vi "Dashboard Main.vi"() -> ()   [LabVIEW 2018]
uses:
  Subsystems/Drive/MotionProfile/StartingPosition.ctl
  Subsystems/Drive/MotionProfile/Path_Decider.ctl
  <vilib>/Utility/miscctls.llb/LVRowAndColumnTypeDef.ctl
  <vilib>/event_ctls.llb/eventvkey.ctl
  <vilib>/Rock Robotics/Network Tables/NT Read Numeric Array.vi
  <vilib>/Rock Robotics/WPI/Dashboard/WPI_DashboardLogging Global.vi
panel:
  in  "Select Auto":string(combo)="Select Autonomous ..."
  out "NT Connection":bool
  out "Camera Perf":string
  in  "Camera Settings":T1={"Frame Rate"=30, "Compression"=30, "Size"=1, "DB Camera Config"=FALSE} {"Frame Rate" scale=1.0..30.0; "Compression" scale=100.0..-1.0; "Size" items=["640x480", "320x240", "160x120"]}
  in  "TCP":refnum<k5>
  out "Robot IP":string
  out "Image Message":string="Timeout in Camera Communications"
  in  "Dashboard Tab":T2(tab)
  out "Mode":T3(ring)=enum."Auto Disabled"
  out "Right Camera Perf":cluster{"Bandwidth (Mbps)":dbl, "FPS":dbl}
  out "Yaw":dbl(graph)
  out "Pitch":dbl(graph)
  out "Roll":dbl(graph)
  out "climbPoweredIRLeft":bool
  out "lineIRRearLeft":bool
  out "climbPoweredIRRight":bool
  out "climbSkidIRRight":bool
  out "climbSkidIRLeft":bool
  out "lineIRFrontLeft":bool
  out "lineIRRearRight":bool
  out "lineIRFrontRight":bool
  out "ClimbRearPosition":dbl
  out "ClimbFrontPosition":dbl
  out "DriveLeftEncoder":dbl
  out "DriveRightEncoder":dbl
  out "HatchPanelDistance":dbl(graph)
  out "DriveIMU":T4(graph)
  out "Sonar":dbl(graph)
  in  "Auto Options":T7={"Starting Position"=enum."Middle L1", "First Score Pos"=enum."7", "Second Score Pos"=enum."5"}
  out "AutoValid?":bool
  in  "Rec Mode":enum32{"Stop", "Record", "Playback"}(radio)
  in  "Camera Settings Right":T1={"Frame Rate"=30, "Compression"=30, "Size"=1, "DB Camera Config"=FALSE} {"Frame Rate" scale=1.0..30.0; "Compression" scale=100.0..-1.0; "Size" items=["640x480", "320x240", "160x120"]}
  in  "Camera Name Right":string(combo)="No Camera Selection"
  out "HatchPanelSwitchA":bool
  out "HatchPanelSwitchB":bool
  out "Match Number":dbl
  out "Replay Number":dbl
  out "Match Type":string
  out "Competion":string
  out "Camera Image Right":T8(plugin-control)
  out "Camera Image":T8(plugin-control)
  in  "DB/String 9":string
  in  "DB/String 8":string
  in  "DB/String 7":string
  in  "DB/String 6":string
  in  "DB/String 5":string
  in  "DB/String 4":string
  in  "DB/String 3":string
  in  "DB/String 2":string
  in  "DB/String 1":string
  in  "DB/String 0":string
  in  "DB/Slider 0":dbl(slide) scale=0.0..5.0
  in  "DB/Slider 1":dbl(slide) scale=0.0..5.0
  in  "DB/Slider 2":dbl(slide) scale=0.0..5.0
  in  "DB/Slider 3":dbl(slide) scale=0.0..5.0
  out "DB/LED 3":bool
  out "DB/LED 2":bool
  out "DB/LED 1":bool
  out "DB/LED 0":bool
  in  "DB/Button 3":bool
  in  "DB/Button 2":bool
  in  "DB/Button 1":bool
  in  "DB/Button 0":bool caption="New Name"
  in  "A PID gains":T9={"proportional gain (Kc)"=0.039, "integral time (Ti, min)"=0.0, "derivative time (Td, min)"=0.0018000000000000004} {"derivative time (Td, min)" format="%.4f"; "integral time (Ti, min)" format="%.4f"; "proportional gain (Kc)" format="%.4f"}
  in  "B PID gains":T9={"proportional gain (Kc)"=0.027999999999999997, "integral time (Ti, min)"=0.0, "derivative time (Td, min)"=0.0018000000000000004} {"derivative time (Td, min)" format="%.4f"; "integral time (Ti, min)" format="%.4f"; "proportional gain (Kc)" format="%.4f"}
  in  "Test Slider":dbl(slide) scale=0.0..100.0 scale format="%#_3g"
  in  "On/Off":bool caption="Solenoid"
  in  "Test Name":u16(ring) items=["Select the test to run..."]
  in  "Test Tree":string(tree)
  in  "Motor":cluster{"Value":dbl, "Enable":bool} {"Value" scale=-1.0..1.0 scale format="%#_3g"}
  out "Progress":T10 {"Test Progress" scale=0.0..100.0}
  in  "Rev/Fwd":cluster{"Forward":bool, "Reverse":bool}
  in  "Test Ring":u16(ring) items=["Monochrome", "Color"]
  out "Cmd Status":string
  in  "Execute Command":bool
  in  "Command Params":string[][](table)
  in  "Command Selection":i32(listbox)
  in  "CheckList":i32(listbox)
  out "Tree":string(tree)
  out "Background":bool
  in  "Camera Name":string(combo)="No Camera Selection"
  # "HW"
  # "HW"
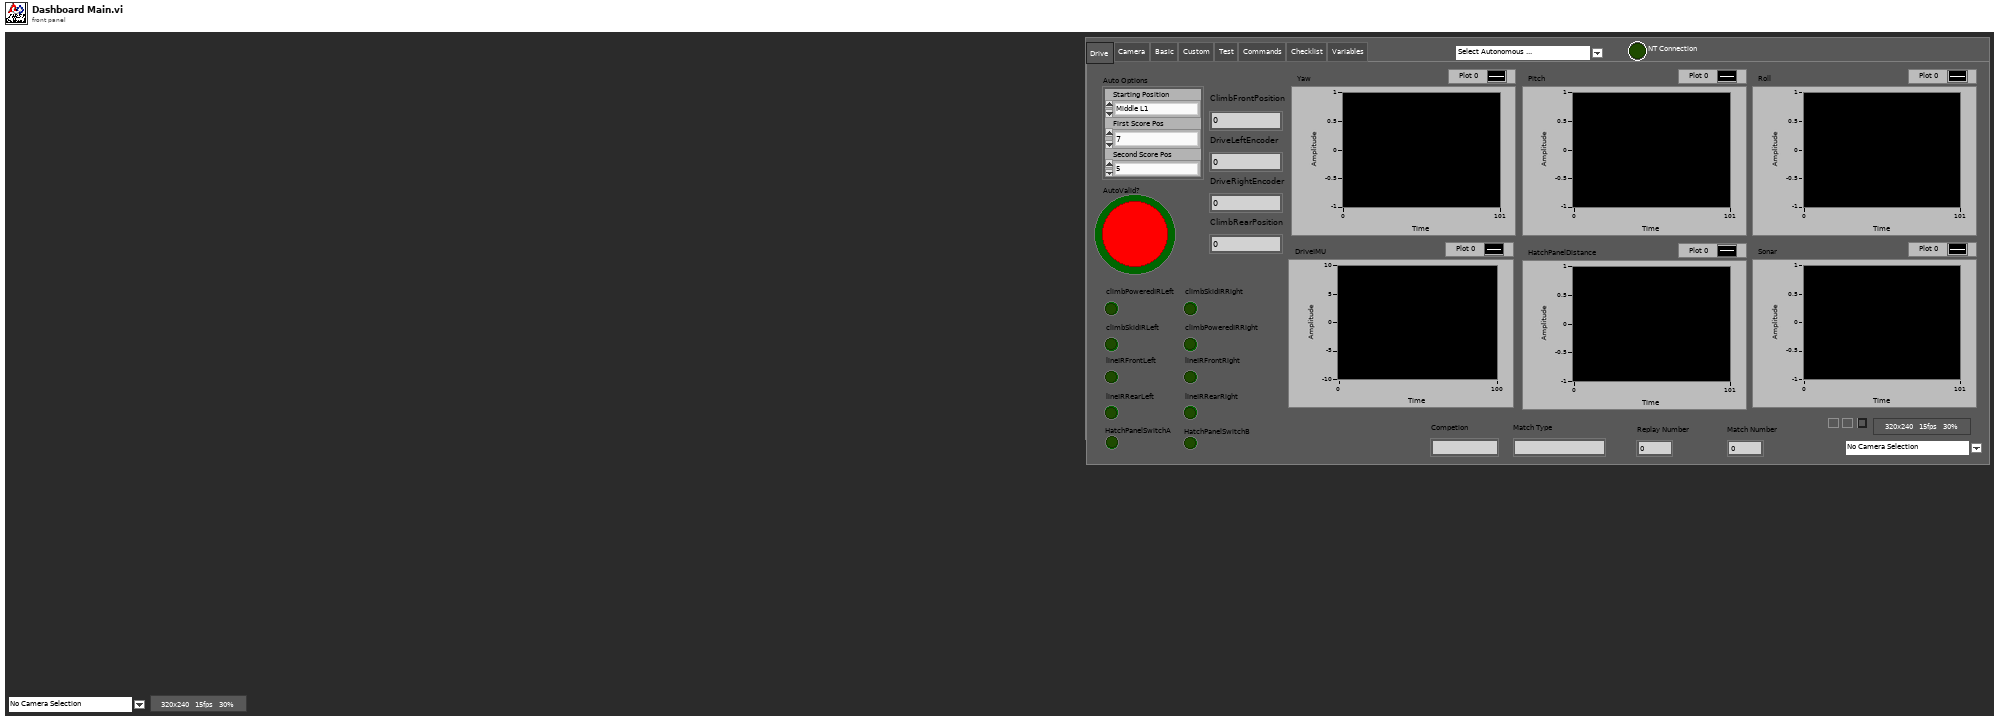
[diagram p1: front panel]
types:
  T1 = cluster{"Frame Rate":i32, "Compression":i32, "Size":u16, "DB Camera Config":bool}
  T2 = enum32{"Drive", "Camera", "Basic", "Custom", "Test", "Commands", "Checklist", "Variables"}
  T3 = enum8{"Tele-Op Disabled", "Tele-Op Enabled", "Auto Disabled", "Auto Enabled", "Test Disabled", "Test Enabled", "Disconnected", "No Code", "E-Stop"}
  T4 = cluster{"Numeric":dbl, "Numeric":dbl, "Numeric":dbl}
  T5 = typedef "StartingPosition.ctl" = enum16{"Left L1 ", "Middle L1", "Right L1", "Left L2", "Right L2", "Don't Move"}
  T6 = typedef "Path_Decider.ctl" = enum16{"1", "2", "3", "4", "5", "6", "7", "8", "Left_Rocket_Front", "Left_Rocket_Rear", "Right_Rocket_Front", "Right_Rocket_Rear"}
  T7 = cluster{"Starting Position":T5, "First Score Pos":T6, "Second Score Pos":T6}
  T8 = typedef "IMAQ Image.ctl" = refnum<image>
  T9 = cluster{"proportional gain (Kc)":dbl, "integral time (Ti, min)":dbl, "derivative time (Td, min)":dbl}
  T10 = cluster{"Test Progress":u8, "Test Progress Text":string}
  T11 = cluster{"Save Path":path, "Interval (s)":dbl, "Keep":i32}
  T12 = typedef "Image Type" = u32
  T13 = cluster{"IDs":cluster{"RPC field ID":u16, "Unique ID":u16}, "String":string}
  T14 = cluster{"Error Strings":string, "Disable Counts":cluster{u16, u16}, "Rail Faults":cluster{u16, u16, u16}, "Robot IP":string, "DB Mode":u8, "Event Info":cluster{"Name":string, "Type":u8, "Number":u16, "Replay":u8}}
  T15 = cluster{"Storage":cluster{"Disk Free":u64, "RAM Block":u32, "RAM free":u32}, "CPU Utilization":cluster{"CPU % ISR":sgl, "CPU % Time Crit":sgl, "CPU % Timed Str":sgl, "CPU % High":sgl, "CPU % Above":sgl, "CPU % Normal":sgl, "CPU % Low":sgl}, "CAN":cluster{"% Bus Utilization":sgl, "Bus Off Cnt":u32, "TX_FIFO Full Cnt":u32, "Receive Error Cnt":u8, "Transmit Error Cnt":u8}, "HID":cluster{"HID Outputs":u32, "Rumble Low":u16, "Rumble High":u16}[]}
  T16 = cluster{"Status bits":cluster{"Test Mode":bool, "Autonomous":bool, "Enabled":bool, "Code Start":bool, "Brownout":bool, "Reserved 2":bool, "Reserved 3":bool, "E-Stop":bool}, "Code Trace":cluster{"Disabled":bool, "TeleOp":bool, "Auto":bool, "Test":bool}, "Controller Type":enum16{"unknown", "cRIO", "roboRio"}, "Code?":enum16{"unknown", "noCode", "code"}, "Battery V":dbl}
  T17 = cluster{"Control Bits":cluster{"TestMode":bool, "Autonomous":bool, "Enabled":bool, "FMS Present":bool, bool, bool, bool, "E-Stop":bool}, "Team Station ":u8, "Countdown":sgl, "Joystick Values":cluster{"Axes":dbl[], "Buttons":bool[], "POVs":i16[]}[]}
  T18 = cluster{"Axes":dbl[], "Buttons":bool[], "POVs":i16[]}[]
  T19 = cluster{"Axes":dbl[], "Buttons":bool[], "POVs":i16[]}
  T20 = cluster{"Camera Image":refnum<vi>, "Dashboard Tab":refnum<vi>, "Background":refnum<vi>, "Rec Mode":refnum<vi>, "Test Slider":refnum<vi>, "On/Off ":refnum<vi>, "Test Ring":refnum<vi>, "Rev/Fwd":refnum<vi>, "Test Name":refnum<vi>, "Motor":refnum<vi>, "Progress":refnum<vi>, "CheckList":refnum<vi>, "Tree":refnum<vi>, "Test Tree":refnum<vi>, "Command Params":refnum<vi>, "Command Selection":refnum<vi>, "Execute Command":refnum<vi>, "Cmd Status":refnum<vi>, "Camera Settings":refnum<vi>, "Camera Name":refnum<vi>, "Camera Perf":refnum<vi>, "Camera Settings Right":refnum<vi>, "Camera Name Right":refnum<vi>, "Camera Image Right":refnum<vi>}
  T21 = cluster{"Global Rectangle":i32[], "Contours":cluster{"Contour Type":u32, "ROI Type":u32, "Points":i32[]}[]}
  T22 = cluster{"Camera Name":string, string, "Saved DB Images Info":cluster{"Save Path":path, "Interval (s)":dbl, "Keep":i32}}
  T23 = cluster{"Camera Name Right":string, string, "Saved DB Images Info":cluster{"Save Path":path, "Interval (s)":dbl, "Keep":i32}}
  T24 = cluster{"Operation":enum16{"Update", "Clear"}, "Color Box":u32}[]
  T25 = typedef "eventvkey.ctl" = enum16{"ASCII", "Enter", "Return", "Shift", "Ctrl", "Alt", "Cmd", "Opt", "Caps", "NumLock", "Clear", "Break", "Up", "Down", "Left", "Right", "Insert", "Delete", "Home", "End", "PageUp", "PageDown", "Escape", "Help", "Pause", "ScrollLock", "F1", "F2", "F3", "F4", "F5", "F6", "F7", "F8", "F9", "F10", "F11", "F12", "F13", "F14", "F15", "F16", "F17", "F18", "F19", "F20", "F21", "F22", "F23", "F24", "Play", "VolumeUp", "VolumeDown", "Mute", "Two Byte Char"}
  T26 = cluster{"Image Size":bool, "Image Type":bool, "Pixel Value":bool, "ROI Information":bool, "Zoom Factor":bool}
  T27 = cluster{"Operation":enum16{"Update", "Clear"}, "Color Box":u32}
  T28 = typedef "LVRowAndColumnTypeDef.ctl" = cluster{"Row":i32, "Column":i32}
  T29 = cluster{"Shift":bool, "Ctrl":bool, "Alt":bool, "Cmd":bool, "Opt":bool}
  T30 = cluster{"Yaw":dbl, "DriveIMU":cluster{"Numeric":dbl, "Numeric":dbl, "Numeric":dbl}, "Sonar":dbl, "Pitch":dbl, "Roll":dbl, "HatchPanelDistance":dbl, "HatchPanelDetect":bool, "climbPoweredIRRight":bool, "climbPoweredIRLeft":bool, "climbSkidIRLeft":bool, "climbSkidIRRight":bool, "lineIRFrontLeft":bool, "lineIRFrontRight":bool, "lineIRRearLeft":bool, "lineIRRearRight":bool, "ClimbFrontPosition":dbl, "ClimbRearPosition":dbl, "DriveRightEncoder":dbl, "DriveLeftEncoder":dbl, "HatchPanelSwitchA":bool, "HatchPanelSwitchB":bool}
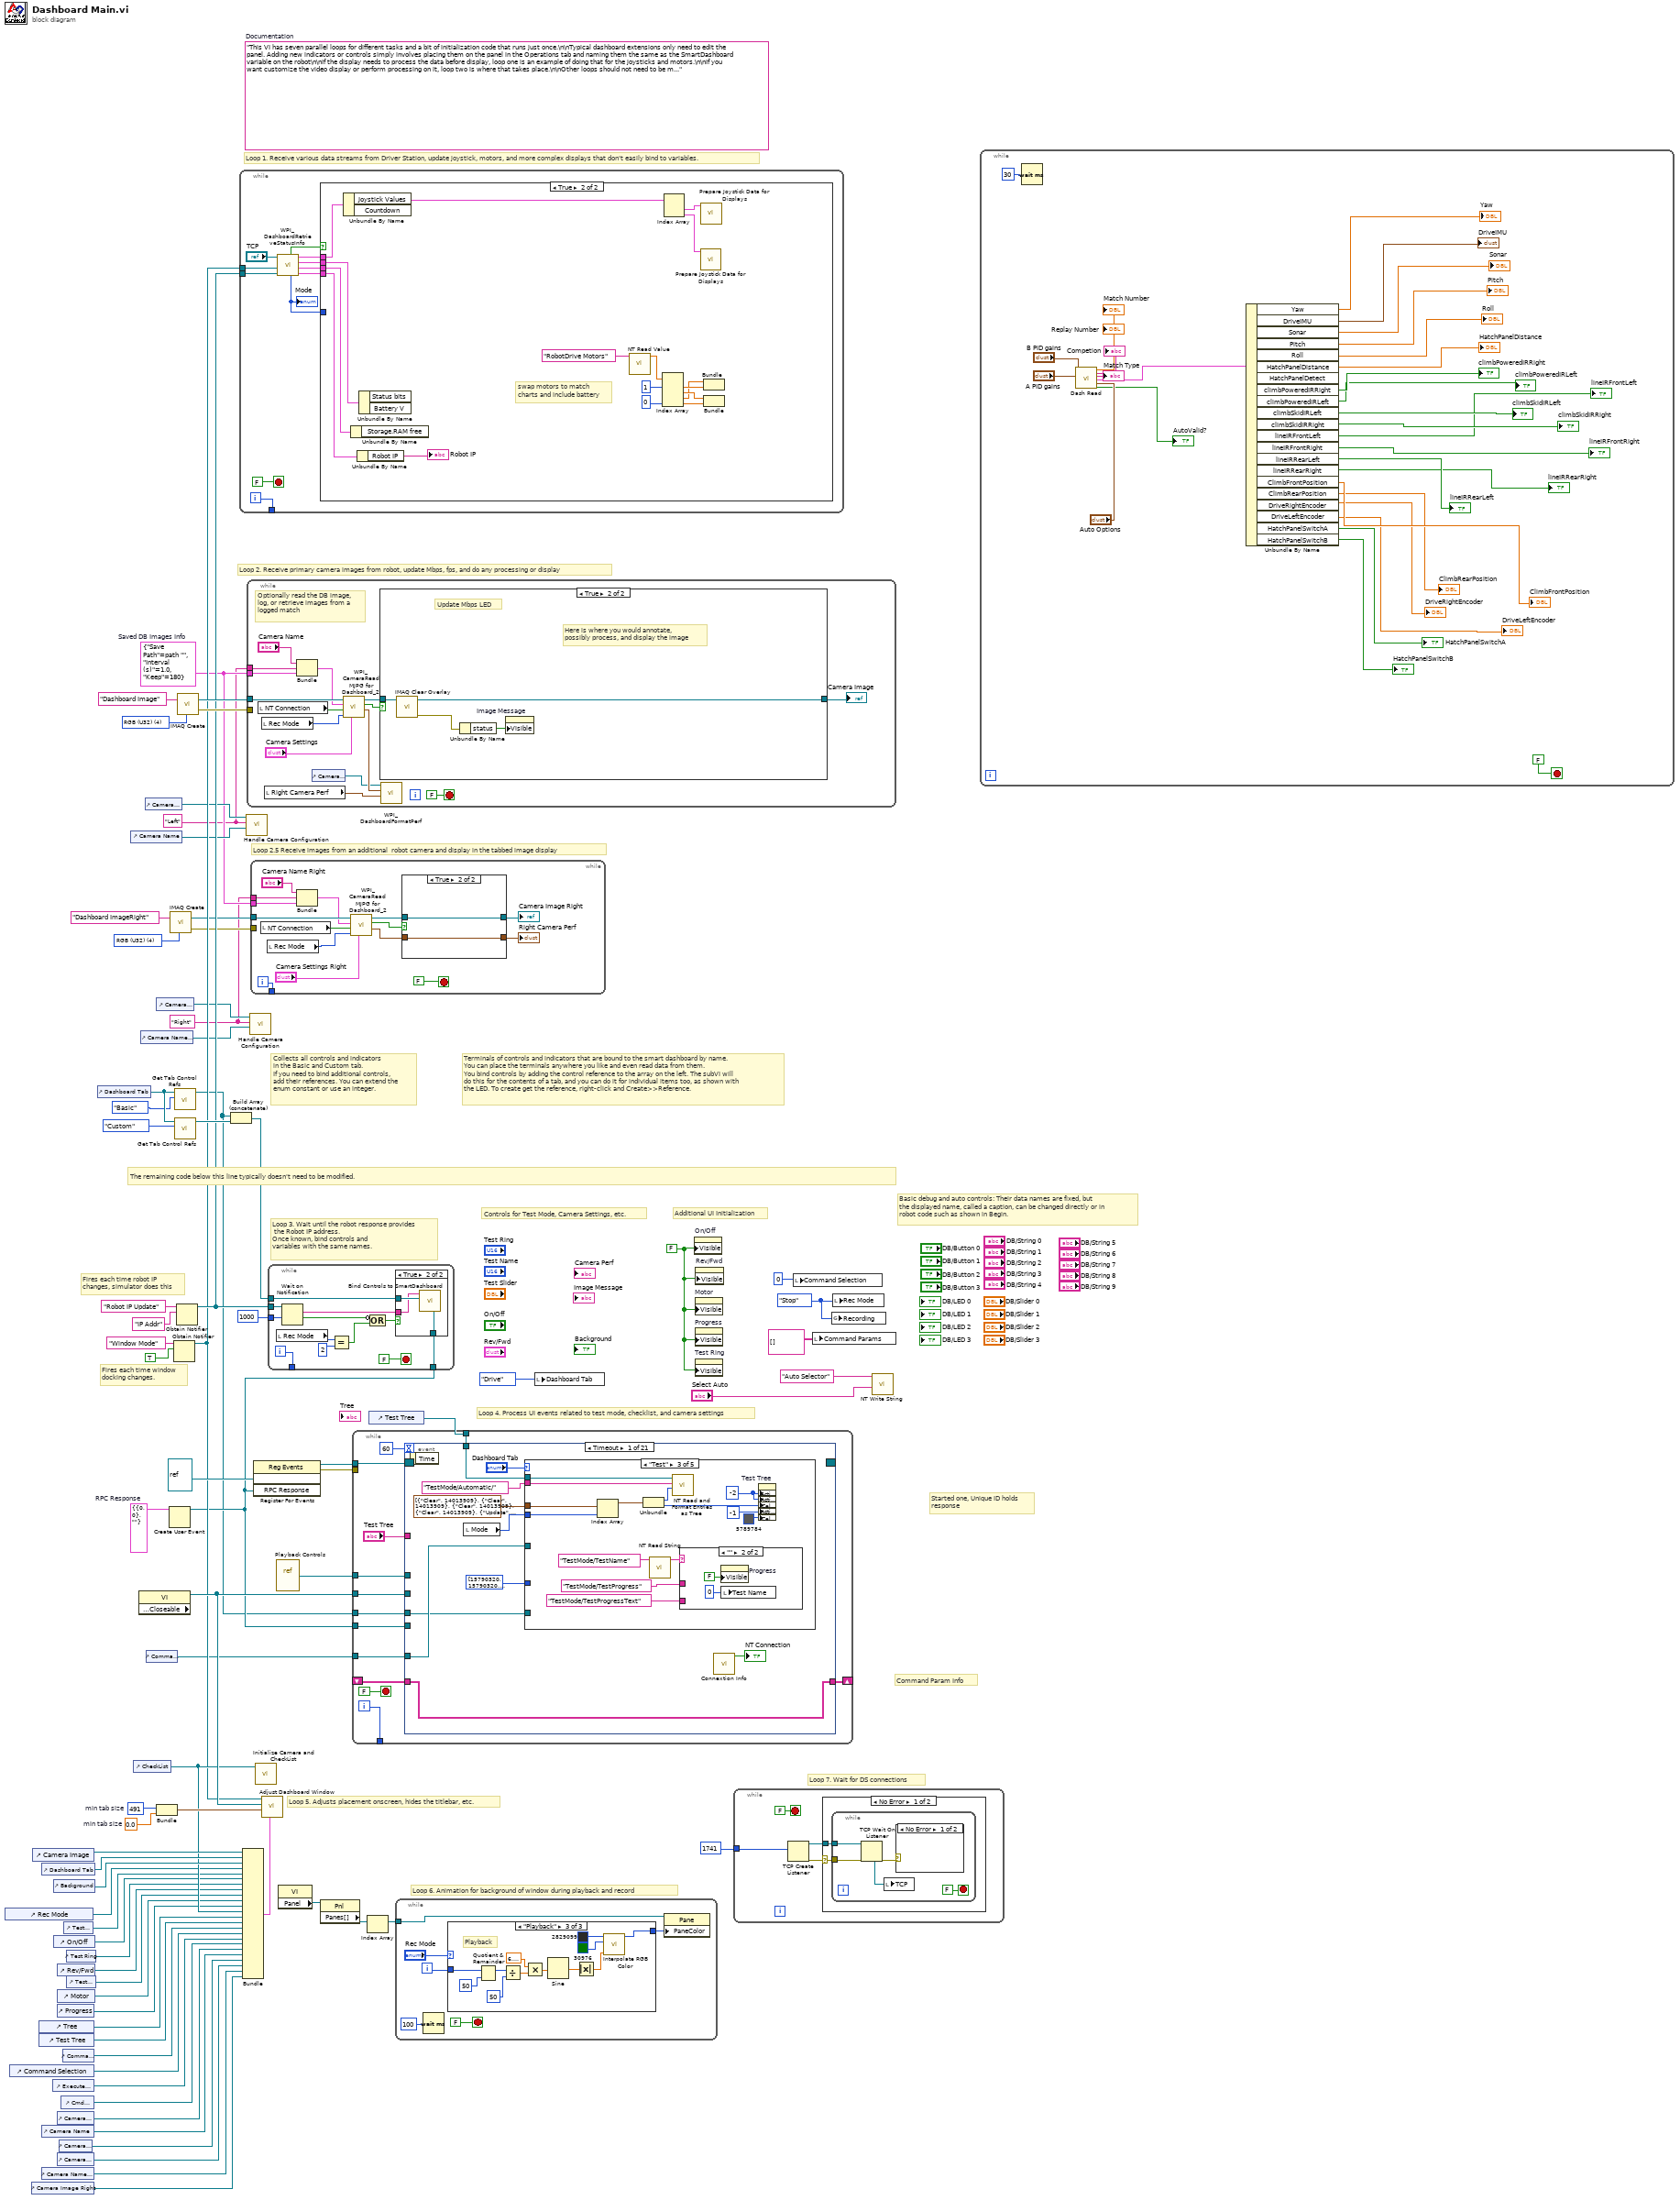
[diagram p0: block diagram]
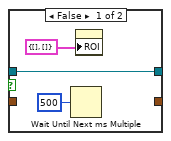
[diagram p2: hidden frame]
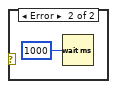
[diagram p3: hidden frame]
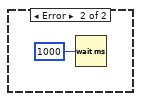
[diagram p4: hidden frame]
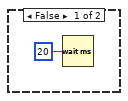
[diagram p5: hidden frame]
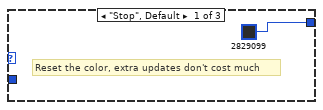
[diagram p6: hidden frame]
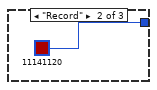
[diagram p7: hidden frame]
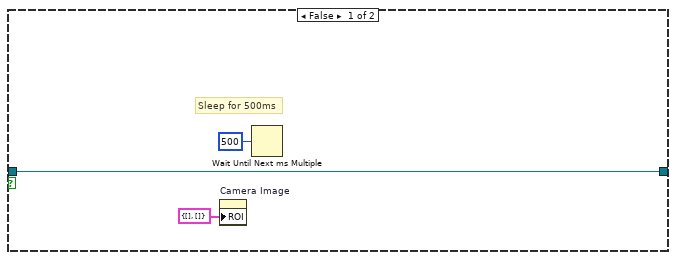
[diagram p9: hidden frame]
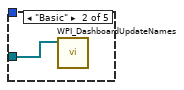
[diagram p11: hidden frame]
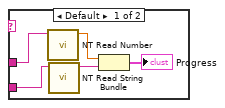
[diagram p12: hidden frame]
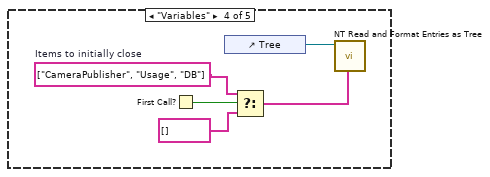
[diagram p13: hidden frame]
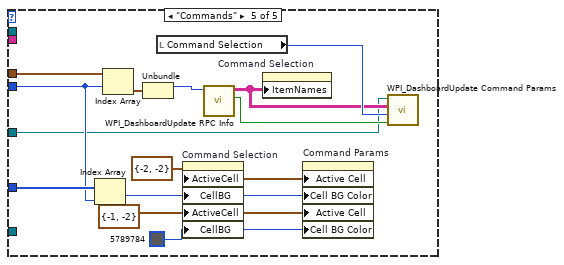
[diagram p14: hidden frame]
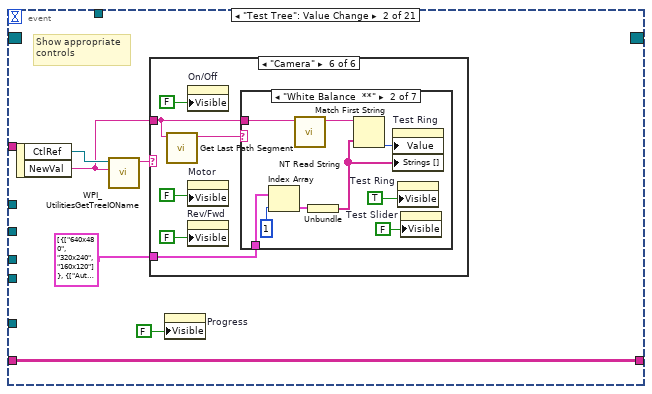
[diagram p15: hidden frame]
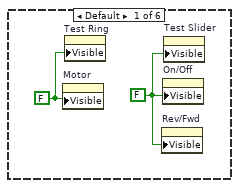
[diagram p16: hidden frame]
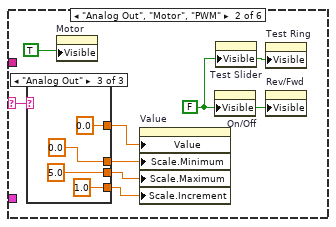
[diagram p17: hidden frame]
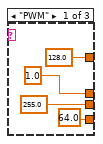
[diagram p18: hidden frame]
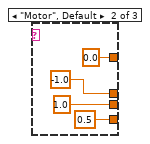
[diagram p19: hidden frame]
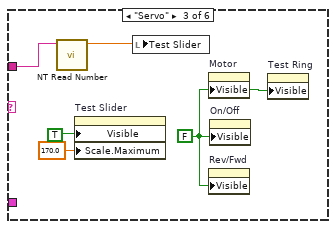
[diagram p20: hidden frame]
diagram:
  w3 = T11 {"Save Path"=path "", "Interval (s)"=1.0, "Keep"=180}  # Saved DB Images Info
  w2 = "Right"
  w1 = "Left"
  w13 = T12 4 items=["Grayscale (U8)", "Grayscale (I16)", "Grayscale (SGL)", "Complex (CSG)", "RGB (U32)", "HSL (U32)", "RGB (U64)"] ("Image Type")
  w29 = T13 {"IDs"={"RPC field ID"=0, "Unique ID"=0}, "String"=""}  # RPC Response
  w52 = 491  # min tab size
  w51 = 0.0  # min tab size
  w59 = enum32{"Stop", "Record", "Playback"}."Stop" ("Rec Mode")
  w36 = FALSE ("Visible")
  (unwired) "This VI has seven parallel loops for different tasks and a bit of initialization code that runs just once.\n\nTypical dashboard extensions only need to edit the panel. Adding new indicators or controls simply involves placing them on the panel in the Operations tab and naming them the same as the SmartDashboard variable on the robot\n\nIf the display needs to process the data before display, loop one is an example of doing that for the joysticks and motors.\n\nIf you want customize the video display or perform processing on it, loop two is where that takes place.\n\nOther loops should not need to be modified. They are pretty standard, and document the task they perform."  # Documentation
  w76 = T12 4 items=["Grayscale (U8)", "Grayscale (I16)", "Grayscale (SGL)", "Complex (CSG)", "RGB (U32)", "HSL (U32)", "RGB (U64)"] ("Image Type")
  # "Loop 2.5 Receive images from an additional  robot camera and display in the tabbed image display"
  # "Command Param Info"
  # "Started one, Unique ID holds\nresponse"
  # "Loop 7. Wait for DS connections"
  # "Basic debug and auto controls: Their data names are fixed, but\nthe displayed name, called a caption, can be changed directly or in\nrobot code such as shown in Begin."
  # "Controls for Test Mode, Camera Settings, etc."
  # "Additional UI Initialization"
  # "Loop 6. Animation for background of window during playback and record"
  # "Fires each time robot IP\nchanges, simulator does this"
  # "Fires each time window\ndocking changes."
  # "Collects all controls and indicators\nin the Basic and Custom tab.\nIf you need to bind additional controls,\nadd their references. You can extend the\nenum constant or use an integer."
  # "The remaining code below this line typically doesn't need to be modified."
  # "Loop 4. Process UI events related to test mode, checklist, and camera settings"
  # "Terminals of controls and indicators that are bound to the smart dashboard by name.\nYou can place the terminals anywhere you like and even read data from them.\nYou bind controls by adding the control reference to the array on the left. The subVI will\ndo this for the contents of a tab, and you can do it for individual items too, as shown with\nthe LED. To create get the reference, right-click and Create>>Reference."
  # "Loop 3. Wait until the robot response provides\n the Robot IP address.\nOnce known, bind controls and\nvariables with the same names."
  # "Loop 5. Adjusts placement onscreen, hides the titlebar, etc."
  # "Loop 1. Receive various data streams from Driver Station, update joystick, motors, and more complex displays that don't easily bind to variables."
  # "Loop 2. Receive primary camera images from robot, update Mbps, fps, and do any processing or display"
  n1 = control-ref of="Rec Mode"() -> (w42:refnum<vi>)
  n2 = control-ref of="Command Selection"() -> (w28:refnum<vi>)
  n3 = control-ref of="Camera Image Right"() -> (w6:refnum<vi>)
  n4 = control-ref of="Camera Image"() -> (w54:refnum<vi>)
  n5 = control-ref of="Tree"() -> (w46:refnum<vi>)
  n6 = control-ref of="Test Tree"() -> (w45:refnum<vi>)
  n7 = control-ref of="Dashboard Tab"() -> (w53:refnum<vi>)
  n8 = control-ref of="Camera Name"() -> (w19:refnum<vi>)
  n9 = control-ref of="Camera Name Right"() -> (w7:refnum<vi>)
  n10 = control-ref of="Execute Command"() -> (w30:refnum<vi>)
  n11 = control-ref of="Background"() -> (w49:refnum<vi>)
  n12 = control-ref of="On/Off"() -> (w40:refnum<vi>)
  n13 = control-ref of="Progress"() -> (w37:refnum<vi>)
  n14 = control-ref of="Camera Settings"() -> (w20:refnum<vi>)
  n15 = control-ref of="Camera Settings Right"() -> (w8:refnum<vi>)
  n16 = control-ref of="Rev/Fwd"() -> (w38:refnum<vi>)
  n17 = control-ref of="Motor"() -> (w43:refnum<vi>)
  n18 = control-ref of="Camera Perf"() -> (w18:refnum<vi>)
  n19 = control-ref of="Cmd Status"() -> (w24:refnum<vi>)
  n20 = control-ref of="Command Params"() -> (w31:refnum<vi>)
  n21 = control-ref of="Test Slider"() -> (w41:refnum<vi>)
  n22 = control-ref of="Test Ring"() -> (w39:refnum<vi>)
  n23 = control-ref of="Test Name"() -> (w44:refnum<vi>)
  n24 = control-ref of="Dashboard Tab"() -> (w57:refnum<vi>)
  n25 = control-ref of="Camera Name"() -> (w21:refnum<vi>)
  n26 = control-ref of="CheckList"() -> (w47:refnum<vi>)
  n27 = property class="VI" props=["Front Panel.Closeable"]() -> (reference out=w58:refnum<vi>)  [unwired: 2 in, 2 out]
  n28 = control-ref of="Camera Name Right"() -> (w9:refnum<vi>)
  n29 = control-ref of="Camera Settings"() -> (w22:refnum<vi>)
  n30 = control-ref of="Command Params"() -> (w23:refnum<vi>)
  n31 = control-ref of="Camera Settings Right"() -> (w10:refnum<vi>)
  n32 = Bundle("min tab size"=w52, "min tab size"=w51) -> (w50:cluster{"min tab size":i32, "min tab size":dbl})  [unwired: 1 in]
  n33 = Create User Event(user event datatype=w29) -> (user event=w25:refnum<user-event>)  [unwired: 1 in, 1 out]
  n34 = call "IMAQ Create"("Image Name"="Dashboard ImageRight", "Image Type"=w13) -> ("New Image"=w12:T8, "error out"=w11:errorcluster)  [unwired: 2 in, 1 out]
  n35 = Obtain Notifier(name (unnamed)="Window Mode", notification data type=TRUE) -> (notifier out=w34:refnum<notifier>)  [unwired: 2 in, 2 out]
  n36 = call <vilib>:"Get Tab Control Refs.vi"("Page Index"=T2."Basic" ("Dashboard Tab"), "TabControl in"=w57) -> ("ControlsOnPage"=w17:refnum<vi>[])  [unwired: 9 in]
  n37 = call <vilib>:"Get Tab Control Refs.vi"("Page Index"=T2."Custom" ("Dashboard Tab"), "TabControl in"=w57) -> ("ControlsOnPage"=w56:refnum<vi>[])  [unwired: 9 in]
  n38 = Obtain Notifier(name (unnamed)="Robot IP Update", notification data type="IP Addr" ("name (unnamed)")) -> (notifier out=w35:refnum<notifier>)  [unwired: 2 in, 2 out]
  n39 = call "IMAQ Create"("Image Name"="Dashboard Image", "Image Type"=w76) -> ("New Image"=w74:T8, "error out"=w73:errorcluster)  [unwired: 2 in, 1 out]
  n40 = Build Array (concatenate)(w17, w56) -> (w55:refnum<vi>[])
  n41 = while {
    tunnel: [w86] -> _
    tunnel: w35 -> [w80]
    tunnel: w34 -> [w77]
    i -> [w86]
    stop <- FALSE stop-if-true
    n42 = call <vilib>:"WPI_DashboardRetrieveStatusInfo.vi"("Binding Refnum"=w80, "Window Mode Notifier"=w77, "TCP Cnx"="TCP") -> ("Power and Errors"=w81:T14, "Robot Metrics"=w84:T15, "Status Info"=w85:T16, "Control Info"=w82:T17, "Robot Mode"=w79:T3, "Process?"=w83:bool)  [unwired: 3 in]
    "Mode" <- w79
    n43 = case shown="True" w83 {
      tunnel: w85 -> [_ w104]
      tunnel: w84 -> [_ w103]
      tunnel: w82 -> [_ w102]
      tunnel: w81 -> [_ w101]
      tunnel: w79 -> [_ _]
      frame False {
        n44 = Wait (ms)(milliseconds to wait=u32 20) -> ()  [unwired: 1 out]
      }
      frame True {
        # "swap motors to match\ncharts and include battery"
        n45 = Unbundle By Name(w102) -> ("Joystick Values"=w94:T18)  [unwired: 1 out]
        n46 = Unbundle By Name(w103) -> ()  [unwired: 1 out]
        n47 = Unbundle By Name(w101) -> ("Robot IP"=→"Robot IP":string)
        n48 = Unbundle By Name(w104) -> ()  [unwired: 2 out]
        n49 = call-poly <vilib>:"NT Read Value.vi"("Name"="RobotDrive Motors") -> ("Numeric Array"=w90:dbl[])  [unwired: 9 in, 1 out]
        n50 = Index Array(array=w90, index #1=1, index #4=0) -> (element #1=w96:dbl, element #2=w97:dbl, element #3=w95:dbl, element #4=w100:dbl)  [unwired: 2 in]
        n51 = Index Array(array=w94) -> (element #1=w93:T19, element #2=w92:T19)  [unwired: 2 in]
        n52 = call "Prepare Joystick Data for Displays.vi"("Joystick Values"=w92) -> ()  [unwired: 8 in, 3 out]
        n53 = call "Prepare Joystick Data for Displays.vi"("Joystick Values"=w93) -> ()  [unwired: 8 in, 3 out]
        n54 = Bundle("Numeric"=w95, "Numeric"=w96) -> ()  [unwired: 1 in, 1 out]
        n55 = Bundle("Numeric"=w97, "Numeric"=w100) -> ()  [unwired: 1 in, 1 out]
      }
    }
  }
  n56 = Bundle("Camera Image"=w54, "Dashboard Tab"=w53, "Background"=w49, "Rec Mode"=w42, "Test Slider"=w41, "On/Off"=w40, "Test Ring"=w39, "Rev/Fwd"=w38, "Test Name"=w44, "Motor"=w43, "Progress"=w37, "CheckList"=w47, "Tree"=w46, "Test Tree"=w45, "Command Params"=w31, "Command Selection"=w28, "Execute Command"=w30, "Cmd Status"=w24, "Camera Settings"=w20, "Camera Name"=w19, "Camera Perf"=w18, "Camera Settings Right"=w8, "Camera Name Right"=w7, "Camera Image Right"=w6) -> (w48:T20)  [unwired: 1 in]
  n57 = call "Handle Camera Configuration.vi"("CameraNameRef"=w21, "Display Name"=w1, "ClusterRef"=w22) -> ()  [unwired: 9 in]
  n58 = while {
    tunnel: w74 -> [w118]
    tunnel: w73 -> [_]
    tunnel: w3 -> [w111]
    tunnel: w1 -> [w108]
    stop <- FALSE stop-if-true
    # "Optionally read the DB image,\nlog, or retrieve images from a\nlogged match"
    n59 = local read "NT Connection"() -> (w112:bool)
    n60 = local read "Rec Mode"() -> (w115:enum32{"Stop", "Record", "Playback"})
    n61 = local read "Right Camera Perf"() -> (w106:cluster{"Bandwidth (Mbps)":dbl, "FPS":dbl})
    n62 = Bundle("Camera Name"="Camera Name", w108, "Saved DB Images Info"=w111) -> (w110:T22)  [unwired: 1 in]
    n63 = control-ref of="Camera Perf"() -> (w105:refnum<vi>)
    n64 = call <vilib>:"WPI_CameraRead MJPG for Dashboard_2.vi"("Camera Settings"="Camera Settings", "Rec Mode"=w115, "NT Connection"=w112, "Capture Info"=w110, "Image in"=w118) -> ("perf info"=w107:cluster{"Bandwidth (Mbps)":dbl, "fps":dbl}, "Active"=w116:bool, "Image\\ out"=w117:T8)  [unwired: 4 in]
    n65 = case shown="True" w116 {
      tunnel: w117 -> [w121 w124]
      tunnel: [w121 w123] -> w113
      frame False {
        # "Sleep for 500ms"
        n66 = property on="Camera Image" class="ImageControl"("ROI"=T21 {"Global Rectangle"=[], "Contours"=[]}) -> ()  [unwired: 2 in, 2 out]
        n67 = Wait Until Next ms Multiple(millisecond multiple=u32 500) -> ()  [unwired: 1 out]
      }
      frame True {
        # "Here is where you would annotate,\npossibly process, and display the image"
        # "Update Mbps LED"
        n68 = call "IMAQ Clear Overlay"("Image"=w124) -> ("error out"=w125:errorcluster, "Image Out"=w123:T8)  [unwired: 2 in, 7 out]
        n69 = Unbundle By Name(w125) -> ("status"=w126:bool)
        n70 = property on="Image Message" class="Str"("Visible"=w126) -> ()  [unwired: 2 in, 2 out]
      }
    }
    "Camera Image" <- w113
    n71 = call <vilib>:"WPI_DashboardFormatPerf.vi"("Right Camera Perf"=w106, "Performance"=w107, "String in"=w105) -> ()  [unwired: 9 in]
  }
  n72 = call "Handle Camera Configuration.vi"("CameraNameRef"=w9, "Display Name"=w2, "ClusterRef"=w10) -> ()  [unwired: 9 in]
  n73 = while {
    tunnel: w12 -> [w141]
    tunnel: w11 -> [_]
    tunnel: [w136] -> _
    tunnel: w3 -> [w132]
    tunnel: w2 -> [w129]
    i -> [w136]
    stop <- FALSE stop-if-true
    n74 = local read "NT Connection"() -> (w133:bool)
    n75 = local read "Rec Mode"() -> (w140:enum32{"Stop", "Record", "Playback"})
    n76 = Bundle("Camera Name Right"="Camera Name Right", w129, "Saved DB Images Info"=w132) -> (w131:T23)  [unwired: 1 in]
    n77 = call <vilib>:"WPI_CameraRead MJPG for Dashboard_2.vi"("Camera Settings"="Camera Settings Right", "Rec Mode"=w140, "NT Connection"=w133, "Capture Info"=w131, "Image in"=w141) -> ("perf info"=w127:cluster{"Bandwidth (Mbps)":dbl, "fps":dbl}, "Active"=w135:bool, "Image\\ out"=w138:T8)  [unwired: 4 in]
    n78 = case shown="True" w135 {
      tunnel: w138 -> [w143 w146]
      tunnel: [w143 w146] -> w134
      tunnel: [_ w145] -> w128
      tunnel: w127 -> [_ w145]
      frame False {
        n79 = Wait Until Next ms Multiple(millisecond multiple=u32 500) -> ()  [unwired: 1 out]
        n80 = property on="Camera Image Right" class="ImageControl"("ROI"=T21 {"Global Rectangle"=[], "Contours"=[]}) -> ()  [unwired: 2 in, 2 out]
      }
      frame True {
      }
    }
    "Camera Image Right" <- w134
    "Right Camera Perf" <- w128
  }
  n81 = register-events(refnum<vi> refnum, w25) -> (reference out=w63:refnum<event-registration>, error out=w62:errorcluster)  [unwired: 2 in]
  n82 = call "Initialize Camera and CheckList.vi"("ListBox in"=w47) -> ()  [unwired: 11 in]
  n83 = call "Adjust Dashboard Window.vi"("Sizing Refnums"=w48, "Size Constraints"=w50, "VI"=w58, "WIn Mode"=w34) -> ()  [unwired: 8 in]
  n84 = while {
    tunnel: w55 -> [w158]
    tunnel: w35 -> [w156]
    tunnel: [w154] -> _
    tunnel: u32 1000 ("milliseconds to wait") -> [w153]
    tunnel: w25 -> [w147]
    i -> [w154]
    stop <- FALSE stop-if-true
    n85 = local read "Rec Mode"() -> (w149:enum32{"Stop", "Record", "Playback"})
    n86 = Wait on Notification(notifier=w156, timeout in ms (-1)=w153) -> (notification=w155:string, timed out?=w151:bool)  [unwired: 2 in, 2 out]
    n87 = Equal?(x=w149, y=u16 2 ("Rec Mode")) -> (x = y?=w150:bool)
    n88 = Compound Arithmetic op=OR(invert w151, w150) -> (w152:bool)
    n89 = case shown="True" w152 {
      tunnel: w158 -> [_ w161]
      tunnel: w155 -> [_ w160]
      tunnel: w147 -> [_ w159]
      frame False {
      }
      frame True {
        n90 = call <vilib>:"Bind Controls to SmartDashboard.vi"("RPC ref"=w159, "Bound Control Refs"=w161, "Server IP Address"=w160) -> ()  [unwired: 9 in]
      }
    }
  }
  n91 = vi-ref "Playback Controls.vi"() -> (w64:refnum<vi>)
  n92 = property class="VI"() -> ("Panel"=w66:refnum<vi>)  [unwired: 2 in, 2 out]
  n93 = property class="Pnl"(reference=w66) -> ("Panes[]"=w67:refnum<vi>[])  [unwired: 1 in, 2 out]
  n94 = Index Array(array=w67) -> (element=w65:refnum<vi>)  [unwired: 1 in]
  n95 = control-ref of="Test Tree"() -> (w68:refnum<vi>)
  n96 = while {
    tunnel: [w171] -> _
    tunnel: w68 -> [w170]
    tunnel: w64 -> [w169]
    tunnel: w63 -> [w168]
    tunnel: w62 -> [_]
    tunnel: w58 -> [w167]
    tunnel: w25 -> [w166]
    tunnel: w23 -> [w165]
    shift-right: [w164] -> _
    shift-left: _ -> [w163]
    tunnel: w17 -> [w162]
    i -> [w171]
    stop <- FALSE stop-if-true
    n97 = event shown="[0] Timeout" {
      selector: w168 -> [_ _ _ _ _ _ _ _ _ _ _ _ _ _ _ _ _ _ _ _ _]
      dyn-events: [_ _ _ _ _ _ _ _ _ _ _ _ _ _ _ _ w431 _ _ _ _] -> _
      timeout: u32 60 ("milliseconds to wait") -> [_ _ _ _ _ _ _ _ _ _ _ _ _ _ _ _ _ _ _ _ _]
      tunnel: w170 -> [w183 _ _ _ _ _ _ _ _ _ _ _ _ _ _ _ _ _ _ _ _]
      tunnel: "Test Tree" -> [_ _ _ _ _ _ _ _ _ _ _ w398 w406 w408 w412 w420 _ _ _ _ _]
      tunnel: w169 -> [_ _ _ _ _ _ _ _ _ _ _ _ _ _ _ _ w433 _ w451 _ _]
      tunnel: w167 -> [_ _ _ _ _ _ _ _ _ _ _ _ _ _ _ _ w429 _ _ _ _]
      tunnel: w166 -> [_ _ _ _ _ _ _ _ _ _ _ _ _ _ _ _ w427 _ _ _ _]
      tunnel: w165 -> [w178 _ _ _ _ _ w349 _ _ _ _ _ _ _ _ _ _ _ _ _ _]
      tunnel: [w177 w226 w328 w333 w342 w346 w347 w356 w366 w373 w385 w397 w404 w407 w411 w419 w426 w446 w448 w452 w465] -> w164
      tunnel: w163 -> [w177 w226 w328 w333 w342 w346 w347 _ _ w373 w385 w397 w404 w407 w411 w419 w426 w446 w448 w452 w465]
      tunnel: w162 -> [w175 _ _ _ _ _ _ _ _ _ _ _ _ _ _ _ _ _ _ _ _]
      event Timeout {
        n98 = event-data() -> ()  [unwired: 1 in, 1 out]
        n99 = local read "Mode"() -> (w180:T3)
        n100 = case shown="\"Test\"" "Dashboard Tab" {
          tunnel: w183 -> [_ _ w199 _ _]
          tunnel: "TestMode/Automatic/" ("Name Pattern") -> [_ _ w198 _ _]
          tunnel: T24 [{"Operation"=enum."Clear", "Color Box"=14013909}, {"Operation"=enum."Clear", "Color Box"=14013909}, {"Operation"=enum."Clear", "Color Box"=14013909}, {"Operation"=enum."Clear", "Color Box"=14013909}, {"Operation"=enum."Update", "Color Box"=14013909}, {"Operation"=enum."Update", "Color Box"=16777215}, {"Operation"=enum."Clear", "Color Box"=14013909}, {"Operation"=enum."Clear", "Color Box"=14013909}, {"Operation"=enum."Clear", "Color Box"=14013909}] -> [_ _ w191 _ w219]
          tunnel: w180 -> [_ _ w190 _ w218]
          tunnel: u32[] [15790320, 15790320, 15790320, 15790320, 16777215, 16777215, 15790320, 15790320, 15790320] -> [_ _ _ _ w224]
          tunnel: w178 -> [_ _ _ _ w212]
          tunnel: w175 -> [_ w185 _ _ _]
          frame "Custom", Default {
          }
          frame "Basic" {
            n101 = call <vilib>:"WPI_DashboardUpdateNames.vi"("Controls on Tab"=w185) -> ()  [unwired: 11 in]
          }
          frame "Test" {
            w197 = -2 ("Active Item:Row Number")
            n102 = Index Array(array=w191, index=w190) -> (element=w192:T27)
            n103 = Unbundle(w192) -> ("Operation"=w193:enum16{"Update", "Clear"}, "Color Box"=w194:u32)
            n104 = call <vilib>:"NT Read String.vi"("Name"="TestMode/TestName") -> ("String"=w188:string)  [unwired: 9 in, 1 out]
            n105 = call <vilib>:"NT Read and Format Entries as Tree.vi"("Operation"=w193, "Name Pattern"=w198, "Tree Refnum"=w199) -> ()  [unwired: 7 in, 2 out]
            n106 = case shown="\"\"" w188 {
              tunnel: "TestMode/TestProgress" ("Name") -> [w201 _]
              tunnel: "TestMode/TestProgressText" ("Name") -> [w200 _]
              frame Default {
                n107 = call <vilib>:"NT Read Number.vi"("Name"=w201) -> ("Numeric"=w202:dbl)  [unwired: 9 in, 1 out]
                n108 = call <vilib>:"NT Read String.vi"("Name"=w200) -> ("String"=w203:string)  [unwired: 9 in, 1 out]
                n109 = Bundle("Numeric"=w202, "String"=w203) -> (→"Progress":cluster{"Numeric":dbl, "String":string})  [unwired: 1 in]
              }
              frame "" {
                n110 = property on="Progress" class="Clust (strict)"("Visible"=FALSE) -> ()  [unwired: 2 in, 2 out]
                n111 = local write "Test Name"(u16 0) -> ()
              }
            }
            n112 = property on="Test Tree" class="Tree (strict)"("Active Item Row Number"=w197, "ActiveColNum"=w197, "CellBG"=w194, "Active Item Row Number"=-1 ("Active Item:Row Number"), "CellBG"=u32 5789784 ("Color Box")) -> ()  [unwired: 2 in, 2 out]
          }
          frame "Variables" {
            w209 = string[] ["CameraPublisher", "Usage", "DB"]  # Items to initially close
            n113 = First Call?() -> (First Call?: T/F=w210:bool)
            n114 = control-ref of="Tree"() -> (w211:refnum<vi>)
            n115 = Select(t=w209, s=w210, f=string[] []) -> (s? t:f=w207:string[])
            n116 = call <vilib>:"NT Read and Format Entries as Tree.vi"("Tags to  Close"=w207, "Tree Refnum"=w211) -> ()  [unwired: 8 in, 2 out]
          }
          frame "Commands" {
            w220 = u32 5789784 ("Color Box")
            w221 = T28 {"Row"=-1, "Column"=-2} ("Active Cell:Active Cell")
            w223 = T28 {"Row"=-2, "Column"=-2} ("Active Cell:Active Cell")
            n117 = Index Array(array=w224, index=w218) -> (element=w222:u32)
            n118 = Index Array(array=w219, index=w218) -> (element=w217:T27)
            n119 = Unbundle(w217) -> ("Operation"=w216:enum16{"Update", "Clear"})  [unwired: 1 out]
            n120 = local read "Command Selection"() -> (w215:i32)
            n121 = property on="Command Selection" class="MCListbox (strict)"("ActiveCell"=w223, "CellBG"=w222, "ActiveCell"=w221, "CellBG"=w220) -> ()  [unwired: 2 in, 2 out]
            n122 = call <vilib>:"WPI_DashboardUpdate RPC Info.vi"("Operation"=w216) -> ("update"=w214:bool, "commands"=w213:string[][])  [unwired: 9 in]
            n123 = property on="Command Selection" class="MCListbox (strict)"("ItemNames"=w213) -> ()  [unwired: 2 in, 2 out]
            n124 = property on="Command Params" class="Tbl (strict)"("Active Cell"=w223, "Cell BG Color"=w222, "Active Cell"=w221, "Cell BG Color"=w220) -> ()  [unwired: 2 in, 2 out]
            n125 = call <vilib>:"WPI_DashboardUpdate Command Params.vi"("Update"=w214, "NewVal"=w215, "Commands"=w213, "Param Tbl"=w212) -> ()  [unwired: 7 in, 1 out]
          }
        }
        n126 = call <vilib>:"Connextion Info.vi"() -> ("Connected"=→"NT Connection":bool)  [unwired: 10 in, 1 out]
      }
      event "Test Tree": Value Change {
        # "Show appropriate\ncontrols"
        n127 = event-data() -> ("CtlRef"=w229:refnum<vi>, "NewVal"=w227:string)  [unwired: 1 in]
        n128 = call <vilib>:"WPI_UtilitiesGetTreeIOName.vi"("NewVal"=w227, "TreeControl in"=w229) -> ("I/O Name"=w230:string)  [unwired: 9 in]
        n129 = case shown="\"Camera\"" w230 {
          selector: w230 -> [_ w237 _ w259 w268 _]
          tunnel: w227 -> [_ _ w256 w258 _ w275]
          tunnel: cluster{string[]}[] [{["640x480", "320x240", "160x120"]}, {["Auto", "Fixed indoor", "Fixed outdoor 1", "Fixed outdoor 2", "Fixed fluorescent 1", "Fixed fluorescent 2", "Hold current"]}, {["Auto", "Flicker-free 50 Hz", "Flicker-free 60 Hz", "Hold current"]}, {["None", "Prioritize frame rate", "Prioritize image quality"]}, {["Monochrome", "Color"]}] -> [_ _ _ _ _ w274]
          frame Default {
            w232 = FALSE ("Visible")
            w231 = FALSE ("Visible")
            n130 = property on="Motor" class="Clust (strict)"("Visible"=w231) -> ()  [unwired: 2 in, 2 out]
            n131 = property on="Test Ring" class="Ring (strict)"("Visible"=w231) -> ()  [unwired: 2 in, 2 out]
            n132 = property on="Rev/Fwd" class="Clust (strict)"("Visible"=w232) -> ()  [unwired: 2 in, 2 out]
            n133 = property on="On/Off" class="Bool (strict)"("Visible"=w232) -> ()  [unwired: 2 in, 2 out]
            n134 = property on="Test Slider" class="Slide (strict)"("Visible"=w232) -> ()  [unwired: 2 in, 2 out]
          }
          frame "Analog Out", "Motor", "PWM" {
            w238 = FALSE ("Visible")
            n135 = case shown="\"Analog Out\"" w237 {
              tunnel: [1.0 ("Value") -1.0 ("Value") 0.0 ("Value")] -> w236
              tunnel: [255.0 ("Value") 1.0 ("Value") 5.0 ("Value")] -> w235
              tunnel: [128.0 ("Value") 0.0 ("Value") 0.0 ("Value")] -> w234
              tunnel: [64.0 ("Value") 0.5 ("Value") 1.0 ("Value")] -> w233
              frame "PWM" {
              }
              frame "Motor", Default {
              }
              frame "Analog Out" {
              }
            }
            n136 = property on="Motor" class="Clust (strict)"("Visible"=TRUE) -> ()  [unwired: 2 in, 2 out]
            n137 = property on="Value" class="Slide (strict)"("Value"=w234, "Scale.Minimum"=w236, "Scale.Maximum"=w235, "Scale.Increment"=w233) -> ()  [unwired: 2 in, 2 out]
            n138 = property on="On/Off" class="Bool (strict)"("Visible"=w238) -> ()  [unwired: 2 in, 2 out]
            n139 = property on="Test Slider" class="Slide (strict)"("Visible"=w238) -> ()  [unwired: 2 in, 2 out]
            n140 = property on="Test Ring" class="Ring (strict)"("Visible"=w238) -> ()  [unwired: 2 in, 2 out]
            n141 = property on="Rev/Fwd" class="Clust (strict)"("Visible"=w238) -> ()  [unwired: 2 in, 2 out]
          }
          frame "Servo" {
            w254 = FALSE ("Visible")
            n142 = call <vilib>:"NT Read Number.vi"("Name"=w256) -> ("Numeric"=w255:dbl)  [unwired: 9 in, 1 out]
            n143 = property on="Test Slider" class="Slide (strict)"("Visible"=TRUE, "Scale.Maximum"=170.0 ("Scale.Range:Maximum")) -> ()  [unwired: 2 in, 2 out]
            n144 = local write "Test Slider"(w255) -> ()
            n145 = property on="Motor" class="Clust (strict)"("Visible"=w254) -> ()  [unwired: 2 in, 2 out]
            n146 = property on="Rev/Fwd" class="Clust (strict)"("Visible"=w254) -> ()  [unwired: 2 in, 2 out]
            n147 = property on="On/Off" class="Bool (strict)"("Visible"=w254) -> ()  [unwired: 2 in, 2 out]
            n148 = property on="Test Ring" class="Ring (strict)"("Visible"=w254) -> ()  [unwired: 2 in, 2 out]
          }
          frame "Relay", "Solenoid" {
            w257 = FALSE ("Visible")
            n149 = property on="Motor" class="Clust (strict)"("Visible"=w257) -> ()  [unwired: 2 in, 2 out]
            n150 = property on="Test Slider" class="Slide (strict)"("Visible"=w257) -> ()  [unwired: 2 in, 2 out]
            n151 = Search and Replace String(input string=w258, search string="/Value  **", replace string="/Direction") -> (result string=w264:string)  [unwired: 5 in, 3 out]
            n152 = property on="Test Ring" class="Ring (strict)"("Visible"=w257) -> ()  [unwired: 2 in, 2 out]
            n153 = call <vilib>:"NT Read String.vi"("Name"=w264) -> ("String"=w262:string)  [unwired: 9 in, 1 out]
            n154 = Equal?(x="Both directions", y=w262) -> (x = y?=w260:bool)
            n155 = Not(x=w260) -> (.not. x?=w261:bool)
            n156 = property on="Rev/Fwd" class="Clust (strict)"("Visible"=w260) -> ()  [unwired: 2 in, 2 out]
            n157 = property on="On/Off" class="Bool (strict)"("Visible"=w261, "Caption.Text"=w259) -> ()  [unwired: 2 in, 2 out]
          }
          frame "Compressor", "Digital Out" {
            w267 = FALSE ("Visible")
            # "Get direction and finish"
            n158 = property on="Motor" class="Clust (strict)"("Visible"=w267) -> ()  [unwired: 2 in, 2 out]
            n159 = property on="Test Slider" class="Slide (strict)"("Visible"=w267) -> ()  [unwired: 2 in, 2 out]
            n160 = property on="Test Ring" class="Ring (strict)"("Visible"=w267) -> ()  [unwired: 2 in, 2 out]
            n161 = property on="On/Off" class="Bool (strict)"("Visible"=TRUE, "Caption.Text"=w268) -> ()  [unwired: 2 in, 2 out]
            n162 = property on="Rev/Fwd" class="Clust (strict)"("Visible"=FALSE) -> ()  [unwired: 2 in, 2 out]
          }
          frame "Camera" {
            n163 = call <vilib>:"Get Last Path Segment.vi"("String in"=w275) -> ("String out"=w276:string)  [unwired: 10 in]
            n164 = property on="On/Off" class="Bool (strict)"("Visible"=FALSE) -> ()  [unwired: 2 in, 2 out]
            n165 = property on="Motor" class="Clust (strict)"("Visible"=FALSE) -> ()  [unwired: 2 in, 2 out]
            n166 = property on="Rev/Fwd" class="Clust (strict)"("Visible"=FALSE) -> ()  [unwired: 2 in, 2 out]
            n167 = case shown="\"White Balance  **\"" w276 {
              tunnel: w275 -> [w282 w291 w300 w309 w318 _ w324]
              tunnel: w274 -> [w280 w288 w297 w306 w315 _ _]
              frame "Size  **" {
                n168 = Index Array(array=w280) -> (element=w279:cluster{string[]})  [unwired: 1 in]
                n169 = call <vilib>:"NT Read String.vi"("Name"=w282) -> ("String"=w281:string)  [unwired: 9 in, 1 out]
                n170 = Unbundle(w279) -> (w277:string[])
                n171 = Match First String(2:w277, 3:w281) -> (0:w278:i32)  [unwired: 1 out]
                n172 = property on="Test Ring" class="Ring (strict)"("Value"=w278, "Strings []"=w277) -> ()  [unwired: 2 in, 2 out]
                n173 = property on="Test Ring" class="Ring (strict)"("Visible"=TRUE) -> ()  [unwired: 2 in, 2 out]
                n174 = property on="Test Slider" class="Slide (strict)"("Visible"=FALSE) -> ()  [unwired: 2 in, 2 out]
              }
              frame "White Balance  **" {
                n175 = Index Array(array=w288, index=1) -> (element=w289:cluster{string[]})
                n176 = call <vilib>:"NT Read String.vi"("Name"=w291) -> ("String"=w290:string)  [unwired: 9 in, 1 out]
                n177 = Unbundle(w289) -> (w286:string[])
                n178 = Match First String(2:w286, 3:w290) -> (0:w285:i32)  [unwired: 1 out]
                n179 = property on="Test Ring" class="Ring (strict)"("Value"=w285, "Strings []"=w286) -> ()  [unwired: 2 in, 2 out]
                n180 = property on="Test Ring" class="Ring (strict)"("Visible"=TRUE) -> ()  [unwired: 2 in, 2 out]
                n181 = property on="Test Slider" class="Slide (strict)"("Visible"=FALSE) -> ()  [unwired: 2 in, 2 out]
              }
              frame "Exposure  **" {
                n182 = Index Array(array=w297, index=2) -> (element=w298:cluster{string[]})
                n183 = call <vilib>:"NT Read String.vi"("Name"=w300) -> ("String"=w299:string)  [unwired: 9 in, 1 out]
                n184 = Unbundle(w298) -> (w294:string[])
                n185 = Match First String(2:w294, 3:w299) -> (0:w295:i32)  [unwired: 1 out]
                n186 = property on="Test Ring" class="Ring (strict)"("Value"=w295, "Strings []"=w294) -> ()  [unwired: 2 in, 2 out]
                n187 = property on="Test Ring" class="Ring (strict)"("Visible"=TRUE) -> ()  [unwired: 2 in, 2 out]
                n188 = property on="Test Slider" class="Slide (strict)"("Visible"=FALSE) -> ()  [unwired: 2 in, 2 out]
              }
              frame "Exposure Priority  **" {
                n189 = Index Array(array=w306, index=3) -> (element=w307:cluster{string[]})
                n190 = call <vilib>:"NT Read String.vi"("Name"=w309) -> ("String"=w308:string)  [unwired: 9 in, 1 out]
                n191 = Unbundle(w307) -> (w303:string[])
                n192 = Match First String(2:w303, 3:w308) -> (0:w304:i32)  [unwired: 1 out]
                n193 = property on="Test Ring" class="Ring (strict)"("Value"=w304, "Strings []"=w303) -> ()  [unwired: 2 in, 2 out]
                n194 = property on="Test Ring" class="Ring (strict)"("Visible"=TRUE) -> ()  [unwired: 2 in, 2 out]
                n195 = property on="Test Slider" class="Slide (strict)"("Visible"=FALSE) -> ()  [unwired: 2 in, 2 out]
              }
              frame "Color Enable  **" {
                n196 = Index Array(array=w315, index=4) -> (element=w316:cluster{string[]})
                n197 = call <vilib>:"NT Read String.vi"("Name"=w318) -> ("String"=w317:string)  [unwired: 9 in, 1 out]
                n198 = Unbundle(w316) -> (w312:string[])
                n199 = Match First String(2:w312, 3:w317) -> (0:w313:i32)  [unwired: 1 out]
                n200 = property on="Test Ring" class="Ring (strict)"("Value"=w313, "Strings []"=w312) -> ()  [unwired: 2 in, 2 out]
                n201 = property on="Test Ring" class="Ring (strict)"("Visible"=TRUE) -> ()  [unwired: 2 in, 2 out]
                n202 = property on="Test Slider" class="Slide (strict)"("Visible"=FALSE) -> ()  [unwired: 2 in, 2 out]
              }
              frame Default {
                n203 = property on="Test Ring" class="Ring (strict)"("Visible"=FALSE) -> ()  [unwired: 2 in, 2 out]
                n204 = property on="Test Slider" class="Slide (strict)"("Visible"=FALSE) -> ()  [unwired: 2 in, 2 out]
              }
              frame "Brightness  **", "Color Level  **", "Compression  **", "FPS  **", "Sharpness  **" {
                n205 = call <vilib>:"NT Read Number.vi"("Name"=w324) -> ("Numeric"=w323:dbl)  [unwired: 9 in, 1 out]
                n206 = local write "Test Slider"(w323) -> ()
                n207 = property on="Test Slider" class="Slide (strict)"("Visible"=TRUE, "Scale.Maximum"=100.0 ("Scale.Range:Maximum")) -> ()  [unwired: 2 in, 2 out]
                n208 = property on="Test Ring" class="Ring (strict)"("Visible"=FALSE) -> ()  [unwired: 2 in, 2 out]
              }
            }
          }
        }
        n209 = property on="Progress" class="Clust (strict)"("Visible"=FALSE) -> ()  [unwired: 2 in, 2 out]
      }
      event "Test Name": Mouse Enter {
        # "Populate the ring with the list of tests"
        n210 = event-data() -> ()  [unwired: 1 in, 1 out]
        n211 = call <vilib>:"NT Read String Array.vi"("Name"="TestMode/TestList") -> ("String Array"=w332:string[])  [unwired: 9 in, 1 out]
        n212 = Build Array (concatenate)("Select the test to run...", w332) -> (w331:string[])
        n213 = property on="Test Name" class="Ring (strict)"("Strings []"=w331) -> ()  [unwired: 2 in, 2 out]
      }
      event "Test Name": Value Change {
        w334 = FALSE ("Visible")
        # "Tell the robot the test name to run"
        n214 = event-data() -> ("NewVal"=w338:u16)  [unwired: 1 in]
        n215 = property on="Test Name" class="Ring (strict)"() -> ("Strings []"=w339:string[])  [unwired: 2 in, 2 out]
        n216 = local write "Progress"(T10 {"Test Progress"=0, "Test Progress Text"=""} ("Progress")) -> ()
        n217 = Index Array(array=w339, index=w338) -> (element=w337:string)
        n218 = call <vilib>:"NT Write String.vi"("String"=w337, "Name"="TestMode/TestName") -> ()  [unwired: 9 in, 1 out]
        n219 = property on="Progress" class="Clust (strict)"("Visible"=TRUE) -> ()  [unwired: 2 in, 2 out]
        n220 = property on="Motor" class="Clust (strict)"("Visible"=w334) -> ()  [unwired: 2 in, 2 out]
        n221 = property on="Test Slider" class="Slide (strict)"("Visible"=w334) -> ()  [unwired: 2 in, 2 out]
        n222 = property on="On/Off" class="Bool (strict)"("Visible"=w334) -> ()  [unwired: 2 in, 2 out]
        n223 = property on="Rev/Fwd" class="Clust (strict)"("Visible"=w334) -> ()  [unwired: 2 in, 2 out]
        n224 = property on="Test Ring" class="Ring (strict)"("Visible"=w334) -> ()  [unwired: 2 in, 2 out]
      }
      event "Select Auto": Mouse Enter {
        # "Populate the combo box with the list of autonomous options"
        n225 = event-data() -> ()  [unwired: 1 in, 1 out]
        n226 = call <vilib>:"NT Read String Array.vi"("Name"="Auto List") -> ("String Array"=w341:string[])  [unwired: 9 in, 1 out]
        n227 = property on="Select Auto" class="CmbBox"("Strings[]"=w341) -> ()  [unwired: 2 in, 2 out]
      }
      event "Select Auto": Value Change {
        # "User modified the Auto Selection. Write to NT variable so robot knows."
        n228 = event-data() -> ("NewVal"=w344:string)  [unwired: 1 in]
        n229 = call <vilib>:"NT Write String.vi"("String"=w344, "Name"="Auto Selector") -> ()  [unwired: 9 in, 1 out]
      }
      event "Command Selection": Value Change {
        # "Get the params and show in table"
        n230 = event-data() -> ("NewVal"=w350:i32)  [unwired: 1 in]
        n231 = property on="Command Selection" class="MCListbox (strict)"() -> ("ItemNames"=w348:string[][])  [unwired: 2 in, 2 out]
        n232 = call <vilib>:"WPI_DashboardUpdate Command Params.vi"("NewVal"=w350, "Commands"=w348, "Param Tbl"=w349) -> ()  [unwired: 8 in, 1 out]
      }
      event "Execute Command": Value Change {
        # "Started one, Unique ID holds\nresponse"
        n233 = event-data() -> ()  [unwired: 1 in, 1 out]
        n234 = property on="Command Selection" class="MCListbox (strict)"() -> ("ItemNames"=w361:string[][])  [unwired: 2 in, 2 out]
        n235 = Index Array(array=w361, index (row)="Command Selection", index (col)=0) -> (element=w359:string)
        n236 = call <vilib>:"Invoke Commands.vi"("Command Params"="Command Params", "Function Name"=w359) -> ("Params"=w355:u8, "Started"=w354:bool)  [unwired: 7 in, 1 out]
        n237 = Array Subset(array="Command Params", length (row)=w355) -> (w356:string[][])  [unwired: 3 in]
        n238 = Select(t="Executing" ("Cmd Status"), s=w354, f="" ("Cmd Status")) -> (s? t:f=→"Cmd Status":string)
      }
      event "Command Selection": Double Click {
        n239 = event-data() -> ("Row"=w369:i32)  [unwired: 1 in]
        n240 = property on="Command Selection" class="MCListbox (strict)"() -> ("ItemNames"=w372:string[][])  [unwired: 2 in, 2 out]
        n241 = local read "Command Params"() -> (w368:string[][])
        n242 = Index Array(array=w372, index (row)=w369, index (col)=0) -> (element=w370:string)
        n243 = call <vilib>:"Invoke Commands.vi"("Command Params"=w368, "Function Name"=w370) -> ("Params"=w367:u8, "Started"=w362:bool)  [unwired: 7 in, 1 out]
        n244 = Array Subset(array=w368, length (row)=w367) -> (w366:string[][])  [unwired: 3 in]
        n245 = Select(t="Executing" ("Cmd Status"), s=w362, f="" ("Cmd Status")) -> (s? t:f=w363:string)
        n246 = local write "Cmd Status"(w363) -> ()
      }
      event "CheckList": Double Click {
        # "Shift clears all"
        # "Update symbols on the listbox"
        n247 = event-data() -> ("PlatMods.Shift"=w374:bool, "Row"=w376:i32)  [unwired: 1 in]
        n248 = case shown="True" w374 {
          tunnel: w376 -> [w380 _]
          tunnel: 1 -> [w379 _]
          frame False {
            n249 = property on="CheckList" class="LstBox (strict)"() -> ("Item Symbols"=w378:i32[])  [unwired: 2 in, 2 out]
            n250 = Replace Array Subset(array=w378, new element=w379, index=w380) -> (w377:i32[])
            n251 = property on="CheckList" class="LstBox (strict)"("Item Symbols"=w377) -> ()  [unwired: 2 in, 2 out]
          }
          frame True {
            w381 = 0 ("Top Row")
            n252 = property on="CheckList" class="LstBox (strict)"() -> ("Number of Rows"=w383:u32)  [unwired: 2 in, 2 out]
            n253 = Initialize Array(0, w383) -> (w382:i32[])
            n254 = property on="CheckList" class="LstBox (strict)"("Top Row"=w381, "Value"=w381, "Item Symbols"=w382) -> ()  [unwired: 2 in, 2 out]
          }
        }
      }
      event "CheckList": Key Down {
        # "Update symbols on the listbox\nLeft and right keys check and uncheck"
        n255 = event-data() -> ("VKey"=w387:T25)  [unwired: 1 in]
        n256 = case shown="\"Left\", \"Right\"" w387 {
          selector: w387 -> [w392 _]
          tunnel: eventvkey."Left" ("VKey") -> [w390 _]
          frame "Left", "Right" {
            n257 = Equal?(x=w390, y=w392) -> (x = y?=w391:bool)
            n258 = Select(t=0, s=w391, f=1) -> (s? t:f=w393:i32)
            n259 = property on="CheckList" class="LstBox (strict)"() -> ("Item Symbols"=w396:i32[])  [unwired: 2 in, 2 out]
            n260 = Replace Array Subset(array=w396, new element=w393, index="CheckList") -> (w395:i32[])
            n261 = property on="CheckList" class="LstBox (strict)"("Item Symbols"=w395) -> ()  [unwired: 2 in, 2 out]
          }
          frame Default {
          }
        }
      }
      event "Motor.Enable": Value Change {
        # "When the test mode otor enable helper is set, update that\ntree row item's value"
        n262 = event-data() -> ("NewVal"=w402:bool)  [unwired: 1 in]
        n263 = Unbundle("Motor") -> ("Value"=w401:dbl)  [unwired: 1 out]
        n264 = Select(t=w401, s=w402, f=0.0) -> (s? t:f=w399:dbl)
        n265 = call <vilib>:"NT Write Number.vi"("Numeric"=w399, "Name"=w398) -> ()  [unwired: 9 in, 1 out]
      }
      event "Test Slider": Value Change {
        # "When the test mode slider helper is set, update that\ntree row item's value"
        n266 = event-data() -> ("NewVal"=w405:dbl)  [unwired: 1 in]
        n267 = call <vilib>:"NT Write Number.vi"("Numeric"=w405, "Name"=w406) -> ()  [unwired: 9 in, 1 out]
      }
      event "On/Off": Value Change {
        # "When the test mode on/off helper value is set, update that\ntree row item's value"
        n268 = event-data() -> ("NewVal"=w410:bool)  [unwired: 1 in]
        n269 = Boolean To (0,1)(Boolean=w410) -> (0, 1=w409:i16)
        n270 = call <vilib>:"NT Write Number.vi"("Numeric"=w409, "Name"=w408) -> ()  [unwired: 9 in, 1 out]
      }
      event "Rev/Fwd": Value Change {
        # "When the test mode helper value for relays is set, update that\ntree row item's value"
        n271 = event-data() -> ("NewVal.Forward"=w418:bool, "NewVal.Reverse"=w417:bool)  [unwired: 1 in]
        n272 = Boolean To (0,1)(Boolean=w418) -> (0, 1=w414:i16)
        n273 = Boolean To (0,1)(Boolean=w417) -> (0, 1=w416:i16)
        n274 = Negate(x=w416) -> (-x=w415:i16)
        n275 = Add(x=w414, y=w415) -> (x+y=w413:i16)
        n276 = call <vilib>:"NT Write Number.vi"("Numeric"=w413, "Name"=w412) -> ()  [unwired: 9 in, 1 out]
      }
      event "Test Ring": Value Change {
        # "When a test mode helper value is selected from the ring,\nset the tree item's variable to the string value"
        n277 = event-data() -> ("NewVal"=w422:u16)  [unwired: 1 in]
        n278 = property on="Test Ring" class="Ring (strict)"() -> ("Strings []"=w423:string[])  [unwired: 2 in, 2 out]
        n279 = Index Array(array=w423, index=w422) -> (element=w421:string)
        n280 = call <vilib>:"NT Write String.vi"("String"=w421, "Name"=w420) -> ()  [unwired: 9 in, 1 out]
      }
      event "Rec Mode": Value Change {
        # "Update globals for recording mode and path to read log from.\nClear when logging and let NetworkTables set path for vision to\nuse."
        n281 = event-data() -> ("NewVal"=w434:enum32{"Stop", "Record", "Playback"})  [unwired: 1 in]
        n282 = global write "WPI_DashboardLogging Global.vi" "Logging Filename"(path "") -> ()
        n283 = global write "WPI_DashboardLogging Global.vi" "Recording"(w434) -> ()
        n284 = case shown="\"Playback\"" w434 {
          tunnel: w433 -> [_ w436 w445]
          tunnel: [_ _ w444] -> w431
          tunnel: [_ _ w443] -> _
          tunnel: w429 -> [_ _ w441]
          tunnel: cluster{i32, i32} {-250, 170} -> [_ _ w440]
          tunnel: [_ _ T26 {"Image Size"=TRUE, "Image Type"=TRUE, "Pixel Value"=TRUE, "ROI Information"=TRUE, "Zoom Factor"=FALSE} ("Image Information Shown:All Elements")] -> w424
          tunnel: [_ _ TRUE ("Zoom Factor")] -> w425
          tunnel: w427 -> [_ _ w437]
          frame Default {
          }
          frame "Stop", "Record" {
            # "Place Window too"
            n285 = invoke class="VI" method="FP.Close"(reference=w436) -> (reference out=w435:refnum<vi>)  [unwired: 2 in, 2 out]
            n286 = invoke class="VI" method="Abort VI"(reference=w435) -> ()  [unwired: 2 in, 3 out]
          }
          frame "Playback" {
            n287 = call "Open Playback Panel.vi"("Offset"=w440, "DB VI Ref"=w441, "Playback in"=w445) -> ("Playback out"=w442:refnum<vi>)  [unwired: 8 in]
            n288 = register-events(w442, w437) -> (reference out=w444:refnum<event-registration>, error out=w443:errorcluster)  [unwired: 2 in]
          }
        }
        n289 = property on="Camera Image Right" class="ImageControl"("Image Information Shown"=w424, "Image Information Visible"=w425) -> ()  [unwired: 2 in, 2 out]
        n290 = property on="Camera Image" class="ImageControl"("Image Information Shown"=w424, "Image Information Visible"=w425) -> ()  [unwired: 2 in, 2 out]
        n291 = call <vilib>:"WPI_DashboardNT Log FieldName Cache.vi"("Operation"=enum16{"Lookup/Add", "Index", "Clear"}."Clear") -> ()  [unwired: 8 in, 3 out]
      }
      event Panel Close {
        w447 = enum32{"Stop", "Record", "Playback"}."Stop" ("Rec Mode")
        # "Playback window has been closed, abort"
        n292 = event-data() -> ()  [unwired: 1 in, 4 out]
        n293 = local write "Rec Mode"(w447) -> ()
        n294 = global write "WPI_DashboardLogging Global.vi" "Recording"(w447) -> ()
      }
      event Panel Close {
        # "Abort playback window and ourself"
        n295 = event-data() -> ()  [unwired: 1 in, 4 out]
        n296 = invoke class="VI" method="FP.Close"(reference=w451) -> (reference out=w450:refnum<vi>)  [unwired: 2 in, 2 out]
        n297 = invoke class="VI" method="Abort VI"(reference=w450) -> (error out=w449:errorcluster)  [unwired: 2 in, 2 out]
        n298 = invoke class="VI" method="Abort VI"(error in=w449) -> ()  [unwired: 2 in, 3 out]
      }
      event User Event {
        n299 = event-data() -> ("IDs"=w458:cluster{"RPC field ID":u16, "Unique ID":u16}, "String"=w457:string)  [unwired: 1 in]
        n300 = Bundle("IDs"=w458, "String"=w457) -> (w456:T13)  [unwired: 1 in]
        n301 = call <vilib>:"Retrieve RPC Response.vi"("RPC Response"=w456) -> ("Output"=w454:string[][])  [unwired: 10 in]
        n302 = Build Array (concatenate)(w452, w454) -> (w453:string[][])
        n303 = local write "Command Params"(w453) -> ()
        n304 = local write "Cmd Status"("" ("Cmd Status")) -> ()
      }
      event "Tree": Double Click {
        n305 = event-data() -> ("PlatMods"=w464:T29, "Tag"=w461:string)  [unwired: 1 in]
        n306 = Unbundle(w464) -> ("Shift"=w463:bool)  [unwired: 4 out]
        n307 = String Subset(string=w461, length (rest)=1 ("length (rest)")) -> (substring=w460:string)  [unwired: 1 in]
        n308 = Not(x=w463) -> (.not. x?=w462:bool)
        n309 = case shown="\"/\"" w460 {
          tunnel: w461 -> [_ w467]
          tunnel: w462 -> [_ w466]
          frame Default {
          }
          frame "/" {
            n310 = call <vilib>:"NT Update Persistence.vi"("Persistence"=w466, "Name"=w467) -> ()  [unwired: 9 in, 1 out]
          }
        }
      }
    }
  }
  n311 = while {
    tunnel: w65 -> [w469]
    i -> [w472]
    stop <- FALSE stop-if-true
    n312 = Wait (ms)(milliseconds to wait=u32 100) -> ()  [unwired: 1 out]
    n313 = case shown="\"Playback\"" "Rec Mode" {
      tunnel: w472 -> [_ _ w487]
      tunnel: [u32 2829099 ("Base Color") u32 11141120 ("Target Color") w476] -> w468
      frame "Stop", Default {
        # "Reset the color, extra updates don't cost much"
      }
      frame "Record" {
      }
      frame "Playback" {
        # "Playback"
        n314 = Quotient & Remainder(x=w487, y=u32 50 ("milliseconds to wait")) -> (x-y*floor(x/y)=w483:u32)  [unwired: 1 out]
        n315 = Divide(x=w483, y=u32 50 ("milliseconds to wait")) -> (x/y=w480:dbl)
        n316 = Multiply(x=6.283185307179586, y=w480) -> (x*y=w485:dbl)
        n317 = Sine(x=w485) -> (sin(x)=w484:dbl)
        n318 = Absolute Value(x=w484) -> (abs(x)=w477:dbl)
        n319 = call "Interpolate RGB Color.vi"("Proportion"=w477, "Target Color"=u32 30976, "Base Color"=u32 2829099) -> ("Result Color"=w476:u32)  [unwired: 8 in]
      }
    }
    n320 = property class="Pane"(reference=w469, "PaneColor"=w468) -> ()  [unwired: 1 in, 2 out]
  }
  n321 = local write "Dashboard Tab"(T2."Drive" ("Dashboard Tab")) -> ()
  n322 = property on="On/Off" class="Bool (strict)"("Visible"=w36) -> ()  [unwired: 2 in, 2 out]
  n323 = property on="Motor" class="Clust (strict)"("Visible"=w36) -> ()  [unwired: 2 in, 2 out]
  n324 = property on="Progress" class="Clust (strict)"("Visible"=w36) -> ()  [unwired: 2 in, 2 out]
  n325 = property on="Test Ring" class="Ring (strict)"("Visible"=w36) -> ()  [unwired: 2 in, 2 out]
  n326 = property on="Rev/Fwd" class="Clust (strict)"("Visible"=w36) -> ()  [unwired: 2 in, 2 out]
  n327 = while {
    tunnel: u16 1741 ("timeout ms (25000)") -> [w489]
    stop <- FALSE stop-if-true
    n328 = TCP Create Listener(10:w489) -> (0:w488:errorcluster, 3:w490:refnum<k5>)  [unwired: 4 in, 1 out]
    n329 = case shown="No Error" w488 {
      selector: w488 -> [w492 _]
      tunnel: w490 -> [w493 _]
      frame No Error {
        n330 = while {
          tunnel: w493 -> [w496]
          tunnel: w492 -> [w495]
          stop <- FALSE stop-if-true
          n331 = TCP Wait On Listener(8:w495, 11:w496) -> (0:w497:errorcluster, 4:w498:refnum<k5>)  [unwired: 2 in, 3 out]
          n332 = local write "TCP"(w498) -> ()
          n333 = case shown="No Error" w497 {
            frame No Error {
            }
            frame Error {
              n334 = Wait (ms)(milliseconds to wait=u32 1000) -> ()  [unwired: 1 out]
            }
          }
        }
      }
      frame Error {
        n335 = Wait (ms)(milliseconds to wait=u32 1000) -> ()  [unwired: 1 out]
      }
    }
  }
  n336 = local write "Command Selection"(u16 0 ("milliseconds to wait")) -> ()
  n337 = local write "Command Params"(string[][] [] ("Command Params")) -> ()
  n338 = global write "WPI_DashboardLogging Global.vi" "Recording"(w59) -> ()
  n339 = local write "Rec Mode"(w59) -> ()
  n340 = call <vilib>:"NT Write String.vi"("String"="Select Auto", "Name"="Auto Selector") -> ()  [unwired: 9 in, 1 out]
  n341 = while {
    stop <- FALSE stop-if-true
    n342 = Wait (ms)(milliseconds to wait=u32 30) -> ()  [unwired: 1 out]
    n343 = call "Dash Read.vi"("A PID gains"="A PID gains", "B PID gains"="B PID gains", "Auto Options"="Auto Options") -> ("Competion"=→"Competion":string, "Replay Number"=→"Replay Number":dbl, "Match Number"=→"Match Number":dbl, "Match Type"=→"Match Type":string, "output cluster"=w527:T30, "AutoValid?"=→"AutoValid?":bool)  [unwired: 11 in]
    n344 = Unbundle By Name(w527) -> ("Yaw"=→"Yaw":dbl, "DriveIMU"=→"DriveIMU":T4, "Sonar"=→"Sonar":dbl, "Pitch"=→"Pitch":dbl, "Roll"=→"Roll":dbl, "HatchPanelDistance"=→"HatchPanelDistance":dbl, "climbPoweredIRRight"=→"climbPoweredIRRight":bool, "climbPoweredIRLeft"=→"climbPoweredIRLeft":bool, "climbSkidIRLeft"=→"climbSkidIRLeft":bool, "climbSkidIRRight"=→"climbSkidIRRight":bool, "lineIRFrontLeft"=→"lineIRFrontLeft":bool, "lineIRFrontRight"=→"lineIRFrontRight":bool, "lineIRRearLeft"=→"lineIRRearLeft":bool, "lineIRRearRight"=→"lineIRRearRight":bool, "ClimbFrontPosition"=→"ClimbFrontPosition":dbl, "ClimbRearPosition"=→"ClimbRearPosition":dbl, "DriveRightEncoder"=→"DriveRightEncoder":dbl, "DriveLeftEncoder"=→"DriveLeftEncoder":dbl, "HatchPanelSwitchA"=→"HatchPanelSwitchA":bool, "HatchPanelSwitchB"=→"HatchPanelSwitchB":bool)  [unwired: 1 out]
  }
